vi "SetTemp.vi"(8 "error in (no error)":errorcluster, 9 "Humid":dbl, 10 "Temp":dbl, 11 "TempChamber Interface in":refnum<class "TempChamber Interface.lvclass">) -> (0 "error out":errorcluster, 2 "Fb":string, 3 "TempChamber Interface out":refnum<class "TempChamber Interface.lvclass">)   [LabVIEW 2018, in "QMH_Class.lvlib" / "Device.lvlib" / "TempChamber Interface.lvclass"]
uses:
  TempChamber Interface.lvclass
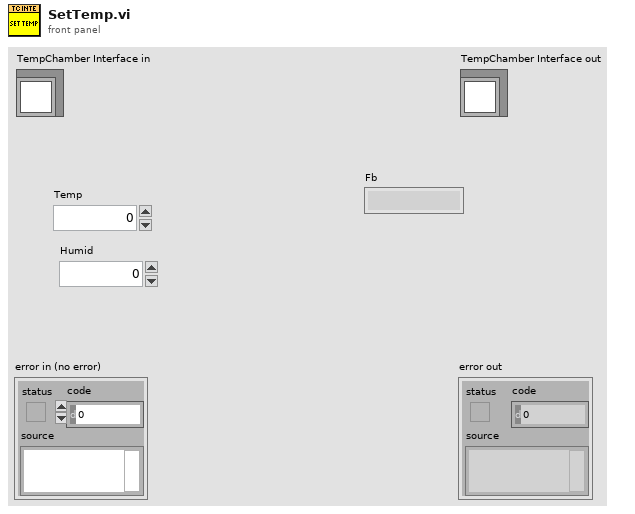
[diagram p1: front panel]
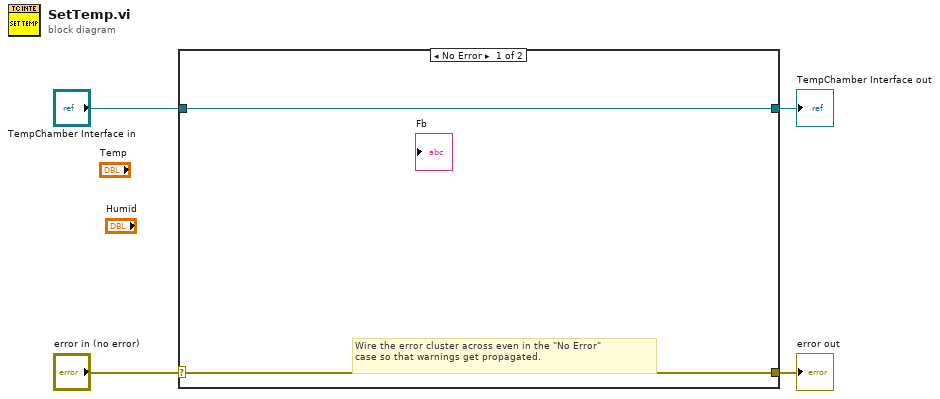
[diagram p0: block diagram]
diagram:
  n1 = case shown="No Error" "error in (no error)" {
    selector: "error in (no error)" -> [w5 w8]
    tunnel: [w5 w8] -> w3
    tunnel: [w6 w7] -> w1
    tunnel: "TempChamber Interface in" -> [w6 w7]
    frame No Error {
      # "Wire the error cluster across even in the \"No Error\"\ncase so that warnings get propagated."
    }
    frame Error {
    }
  }
  "error out" <- w3
  "TempChamber Interface out" <- w1
